vi "dxf提取圆弧坐标点.vi"(11 "字符串":string) -> (3 "输出数组":T1(array[cluster]))   [LabVIEW 2014]
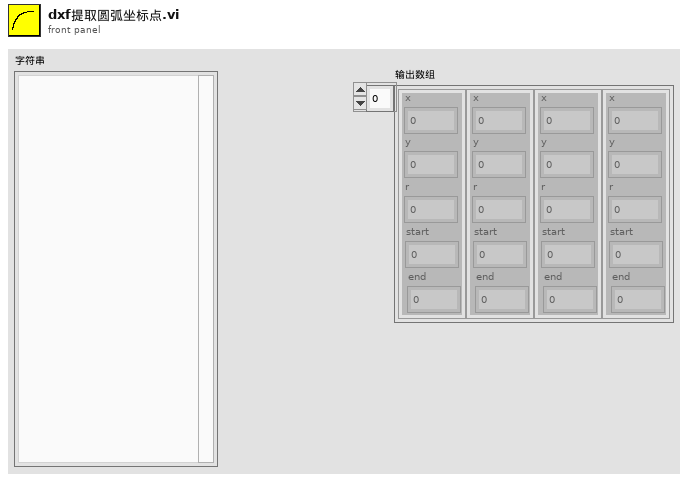
[diagram p1: front panel]
types:
  T1 = cluster{"x":dbl, "y":dbl, "r":dbl, "start":dbl, "end":dbl}[]
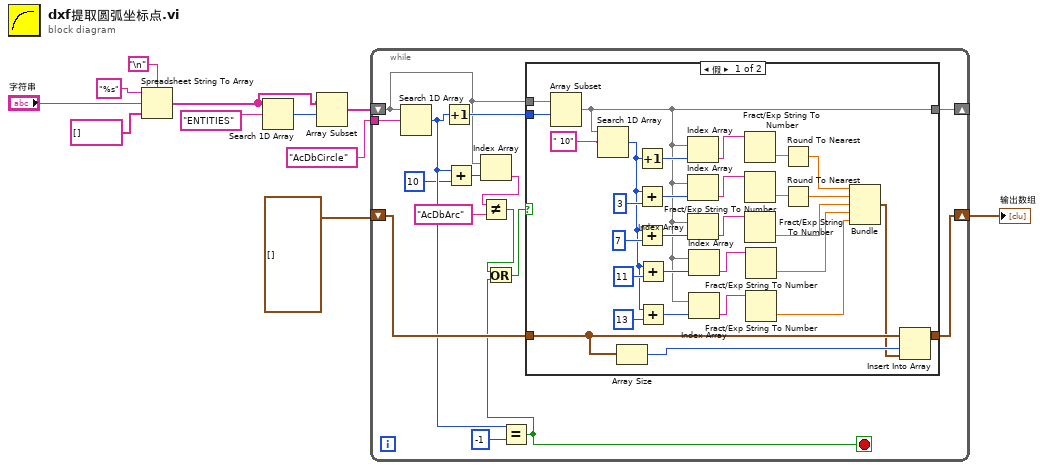
[diagram p0: block diagram]
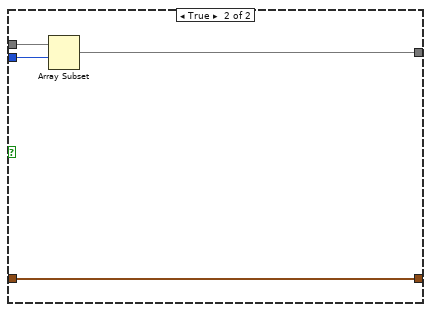
[diagram p2: hidden frame]
diagram:
  n1 = Spreadsheet String To Array(delimiter (Tab)="\n", format string="%s" ("格式字符串"), spreadsheet string="字符串", array type (2D Dbl)=string[] [] ("数组类型(2D Dbl)")) -> (array=w5:string[])
  n2 = Search 1D Array(1D array=w5, element="ENTITIES" ("元素")) -> (index of element=w6:i32)  [unwired: 1 in]
  n3 = Array Subset(array=w5, index=w6) -> (w4:string[])  [unwired: 1 in]
  n4 = while {
    tunnel: "AcDbCircle" ("元素") -> [w26]
    shift-right: [w23] -> _
    shift-left: w4 -> [w20]
    shift-right: [w22] -> w2
    shift-left: cluster{dbl, dbl, dbl, dbl, dbl}[] [] -> [w21]
    stop <- w12 stop-if-true
    n5 = Search 1D Array(1D array=w20, element=w26) -> (index of element=w18:i32)  [unwired: 1 in]
    n6 = Increment(x=w18) -> (x+1=w24:i32)
    n7 = Add(x=w18, y=10) -> (x+y=w19:i32)
    n8 = Index Array(array=w20, index=w19) -> (element=w16:string)
    n9 = Not Equal?(x=w16, y="AcDbArc" ("元素")) -> (x != y?=w13:bool)
    n10 = Equal?(x=w18, y=-1) -> (x = y?=w12:bool)
    n11 = Or(x=w13, y=w12) -> (x .or. y?=w14:bool)
    n12 = case shown="假" w14 {
      tunnel: w24 -> [w56 w57]
      tunnel: [w30 w58] -> w23
      tunnel: [w43 w60] -> w22
      tunnel: w21 -> [w42 w60]
      tunnel: w20 -> [w38 w59]
      frame False {
        n13 = Array Subset(array=w38, index=w56) -> (w30:string[])  [unwired: 1 in]
        n14 = Search 1D Array(1D array=w30, element=" 10") -> (index of element=w27:i32)  [unwired: 1 in]
        n15 = Array Size(array=w42) -> (size(s)=w40:i32)
        n16 = Increment(x=w27) -> (x+1=w55:i32)
        n17 = Add(x=w27, y=i8 3) -> (x+y=w54:i32)
        n18 = Add(x=w27, y=i8 7) -> (x+y=w53:i32)
        n19 = Add(x=w27, y=i8 11) -> (x+y=w35:i32)
        n20 = Add(x=w27, y=i8 13) -> (x+y=w34:i32)
        n21 = Index Array(array=w30, index=w55) -> (element=w50:string)
        n22 = Index Array(array=w30, index=w54) -> (element=w49:string)
        n23 = Index Array(array=w30, index=w53) -> (element=w48:string)
        n24 = Index Array(array=w30, index=w35) -> (element=w32:string)
        n25 = Index Array(array=w30, index=w34) -> (element=w31:string)
        n26 = Fract/Exp String To Number(string=w50) -> (number=w47:dbl)  [unwired: 3 in, 1 out]
        n27 = Fract/Exp String To Number(string=w49) -> (number=w46:dbl)  [unwired: 3 in, 1 out]
        n28 = Fract/Exp String To Number(string=w48) -> (number=w37:dbl)  [unwired: 3 in, 1 out]
        n29 = Fract/Exp String To Number(string=w32) -> (number=w29:dbl)  [unwired: 3 in, 1 out]
        n30 = Fract/Exp String To Number(string=w31) -> (number=w28:dbl)  [unwired: 3 in, 1 out]
        n31 = Round To Nearest(number=w47) -> (nearest integer value=w45:dbl)
        n32 = Round To Nearest(number=w46) -> (nearest integer value=w44:dbl)
        n33 = Bundle(w45, w44, w37, w29, w28) -> (w39:cluster{dbl, dbl, dbl, dbl, dbl})  [unwired: 1 in]
        n34 = Insert Into Array(array=w42, index=w40, new element=w39) -> (w43:cluster{dbl, dbl, dbl, dbl, dbl}[])
      }
      frame True {
        n35 = Array Subset(array=w59, index=w57) -> (w58:string[])  [unwired: 1 in]
      }
    }
  }
  "输出数组" <- w2
